vi "Add alarm to archive.vi"(8 "error in":errorcluster, 11 "Alarm messege":string) -> (0 "error out":errorcluster)   [LabVIEW 2023]
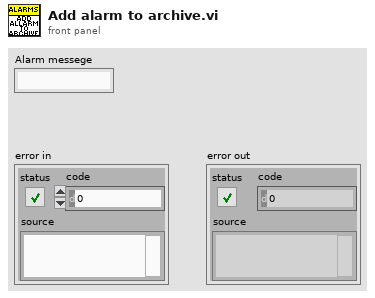
[diagram p1: front panel]
types:
  T1 = enum16{"open", "replace", "create", "open or create", "replace or create", "replace or create with confirmation"}
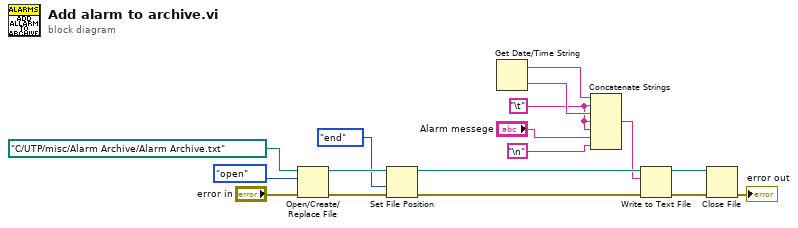
[diagram p0: block diagram]
diagram:
  w1 = "\t"
  n1 = Open/Create/Replace File(file path (use dialog)=path "C:/UTP/misc/Alarm Archive/Alarm Archive.txt", error in="error in", operation (0:open)=T1."open") -> (refnum out=w15:refnum<file>, error out=w13:errorcluster)  [unwired: 3 in, 1 out]
  n2 = Set File Position(refnum=w15, from (0:start)=enum16{"start", "end", "current"}."end", error in=w13) -> (refnum out=w11:refnum<file>, error out=w10:errorcluster)  [unwired: 1 in]
  n3 = Get Date/Time String() -> (date string=w5:string, time string=w4:string)  [unwired: 3 in]
  n4 = Concatenate Strings(w5, w1, w4, w1, w1, "Alarm messege", "\n") -> (w6:string)
  n5 = Write to Text File(file (use dialog)=w11, text=w6, error in=w10) -> (refnum out=w9:refnum<file>, error out=w8:errorcluster)  [unwired: 1 in, 1 out]
  n6 = Close File(refnum=w9, error in=w8) -> (error out=→"error out":errorcluster)  [unwired: 1 out]
